vi "BuildDiffList.vi"(2 "Reference list":string="7161,7162,7163,7164,7165,7166,7167,7168", 3 "Input list":string="7161,7163,7165,7167") -> (0 "Difference list":string)   [LabVIEW 2012]
doc: "Build up a difference list between two input lists.\nThe Input list is a comma-delimited list of entries.\nThe reference list is a comma-delimited list of possible entries.\nThe difference list is a comma-delimited list of entries which exist in the\nreference list but are not in the input list."
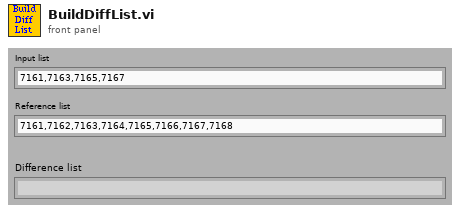
[diagram p1: front panel]
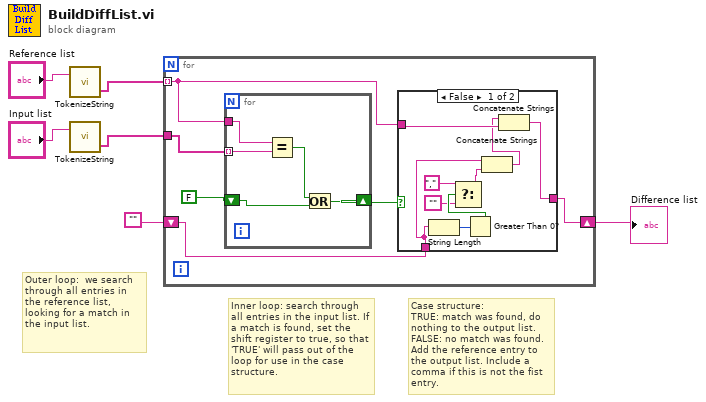
[diagram p0: block diagram]
diagram:
  # "Case structure: \nTRUE: match was found, do nothing to the output list.\nFALSE: no match was found. Add the reference entry to the output list. Include a comma if this is not the fist entry."
  # "Inner loop: search through all entries in the input list. If a match is found, set the shift register to true, so that 'TRUE' will pass out of the loop for use in the case structure."
  # "Outer loop:  we search through all entries in the reference list, looking for a match in the input list."
  n1 = call "TokenizeString.vi"("String to be tokenized"="Reference list") -> ("Output array"=w6:string[])  [unwired: 2 in]
  n2 = call "TokenizeString.vi"("String to be tokenized"="Input list") -> ("Output array"=w5:string[])  [unwired: 2 in]
  n3 = for {
    tunnel: w6 -> [w8] mode=indexing
    tunnel: w5 -> [w11]
    shift-right: [w7] -> w1
    shift-left: "" -> [w9]
    n4 = for {
      tunnel: w8 -> [w23]
      shift-right: [w25] -> w10
      shift-left: FALSE -> [w27]
      tunnel: w11 -> [w24] mode=indexing
      n5 = Equal?(x=w23, y=w24) -> (x = y?=w26:bool)
      n6 = Or(x=w26, y=w27) -> (x .or. y?=w25:bool)
    }
    n7 = case shown="False" w10 {
      tunnel: w9 -> [w15 w22]
      tunnel: w8 -> [w21 _]
      tunnel: [w13 w22] -> w7
      frame False {
        n8 = String Length(string=w15) -> (length=w20:i32)
        n9 = Greater Than 0?(x=w20) -> (x > 0?=w19:bool)
        n10 = Select(t=",", s=w19, f="") -> (s? t:f=w16:string)
        n11 = Concatenate Strings(w15, w16) -> (w14:string)
        n12 = Concatenate Strings(w14, w21) -> (w13:string)
      }
      frame True {
      }
    }
  }
  "Difference list" <- w1
